vi "I2C Read.vi"(8 "error in (no error)":errorcluster, 9 "I2C Address (0x70)":i32=112 format="%x", 10 "Bytes to Read (1)":i32=1, 11 "I2C Task In":T1) -> (0 "error out":errorcluster, 2 "Data":u8[](array[numeric]) format="%x", 3 "I2C Task Out":T1)   [LabVIEW 2017, in "I2C.lvlib"]
doc: "Returns <b>Bytes to Read</b> number of bytes, most significant bit first from the specified address. The I2C address is actually a 7-bit I2C address with an expansion of one 0 at the highest bit."
uses:
  <vilib>/robotics/Protocols/I2C/DAQmx/I2C.lvlib
  <vilib>/robotics/Protocols/I2C/DAQmx/Private/I2C Tasks.ctl
panel:
  # "The I2C address is actually a 7-bit I2C address with an expansion of one 0 at the highest bit."
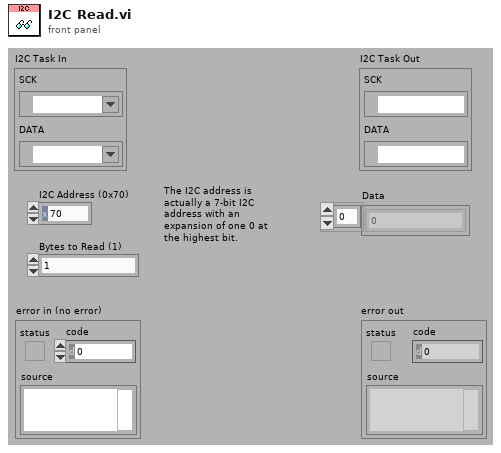
[diagram p1: front panel]
types:
  T1 = typedef "I2C.lvlib/I2C Tasks.ctl" = cluster{"SCK":refnum<k21>, "DATA":refnum<k21>}
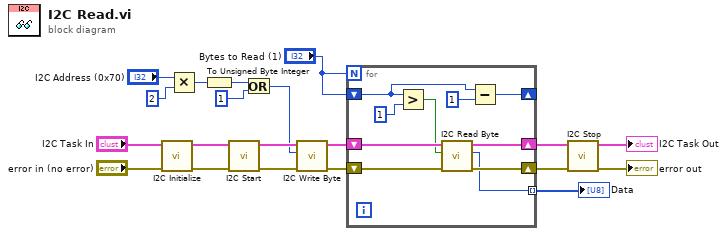
[diagram p0: block diagram]
diagram:
  n1 = call <vilib>:"I2C Initialize.vi"("error in (no error)"="error in (no error)", "I2C Task In"="I2C Task In") -> ("error out"=w17:errorcluster, "I2C Task Out"=w18:T1)  [unwired: 8 in]
  n2 = Multiply(x="I2C Address (0x70)", y=2) -> (x*y=w14:i32)
  n3 = To Unsigned Byte Integer(number=w14) -> (unsigned 8bit integer=w13:u8)
  n4 = call <vilib>:"I2C Start.vi"("error in (no error)"=w17, "I2C Task In"=w18) -> ("error out"=w9:errorcluster, "I2C Task Out"=w11:T1)  [unwired: 8 in]
  n5 = Or(x=w13, y=u8 1) -> (x .or. y?=w10:u8)
  n6 = call <vilib>:"I2C Write Byte.vi"("error in (no error)"=w9, "Data Byte (0x0)"=w10, "I2C Task In"=w11) -> ("error out"=w6:errorcluster, "I2C Task Out"=w7:T1)  [unwired: 6 in, 1 out]
  n7 = for {
    N: "Bytes to Read (1)" -> [_]
    shift-right: [w24] -> _
    shift-left: "Bytes to Read (1)" -> [w26]
    shift-right: [w23] -> w4
    shift-left: w7 -> [w30]
    shift-right: [w22] -> w3
    shift-left: w6 -> [w29]
    tunnel: [w21] -> w5 mode=indexing
    n8 = Greater?(x=w26, y=1) -> (0:w27:bool)
    n9 = call <vilib>:"I2C Read Byte.vi"("error in (no error)"=w29, "Ack? (F:False)"=w27, "I2C Task In"=w30) -> ("error out"=w22:errorcluster, "Data Byte"=w21:u8, "I2C Task Out"=w23:T1)  [unwired: 6 in]
    n10 = Subtract(x=w26, y=1) -> (x-y=w24:i32)
  }
  "Data" <- w5
  n11 = call <vilib>:"I2C Stop.vi"("error in (no error)"=w3, "I2C Task In"=w4) -> ("error out"=→"error out":errorcluster, "I2C Task Out"=→"I2C Task Out":T1)  [unwired: 8 in]
